vi "Analog multimeter producer-consumer.vi"() -> ()   [LabVIEW 2019]
uses:
  Controls/Enum_states.ctl
panel:
  in  "Output channel":T1(ring)
  in  "Input channel":T1(ring)
  in  "Data":bool
  in  "Settings":bool
  out "Message":string
  in  "Stop Button":bool
  out "Terminal GND":bool
  out "Terminal_I":bool
  out "Terminal_V":bool
  in  "Signal":dbl(knob) scale=0.0..1000.0
  in  "Zero instrument":dbl(knob) scale=-1.0..1.0
  in  "Zero resistance":dbl(knob) scale=-1.0..1.0
  in  "Selector":i32(knob)=10 min=0 max=20 step=1 scale=0.0..20.0
  out "Main indicator":dbl(knob) scale=0.0..1000.0
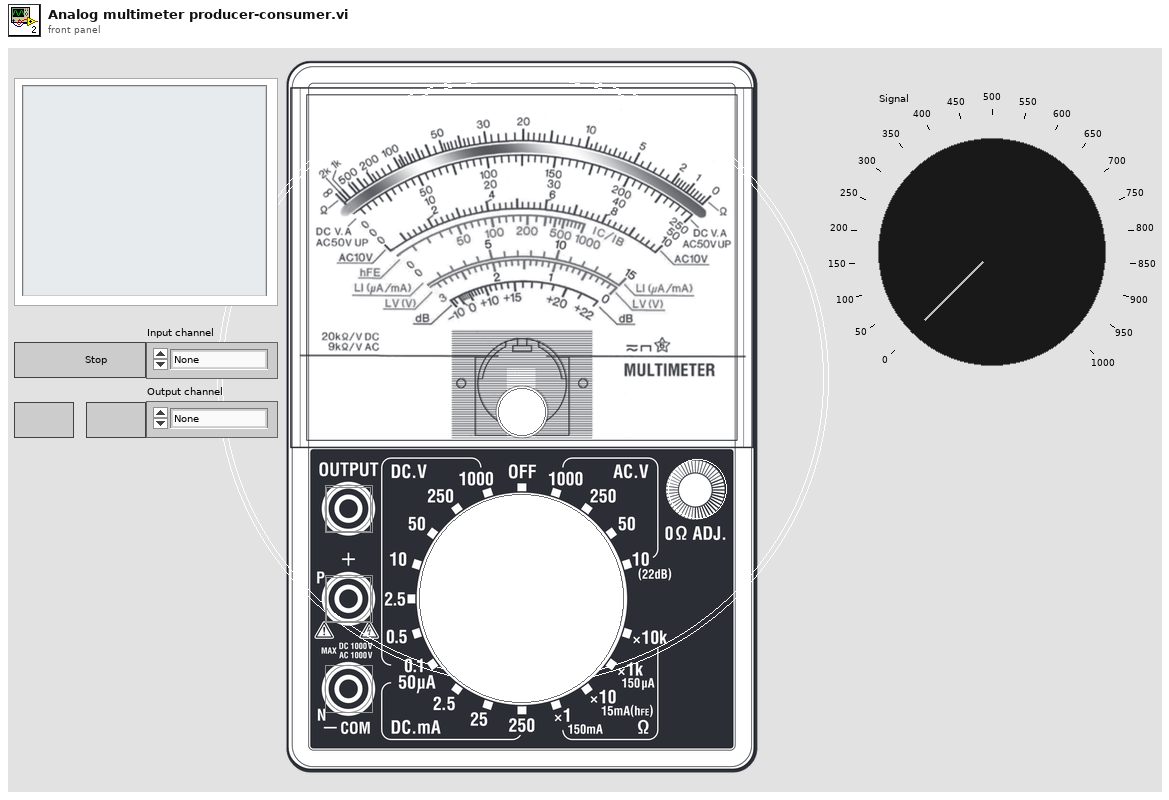
[diagram p1: front panel]
types:
  T1 = enum16{"None", "CH 1", "CH 2", "CH 3", "CH 4", "CH 5", ""}
  T2 = typedef "Enum_states.ctl" = enum16{"Initialize", "Run", "Load", "Stop"}
  T3 = cluster{"Main indicator":dbl, "Terminal_V":bool, "Terminal_I":bool, "Terminal GND":bool, "Message":string}
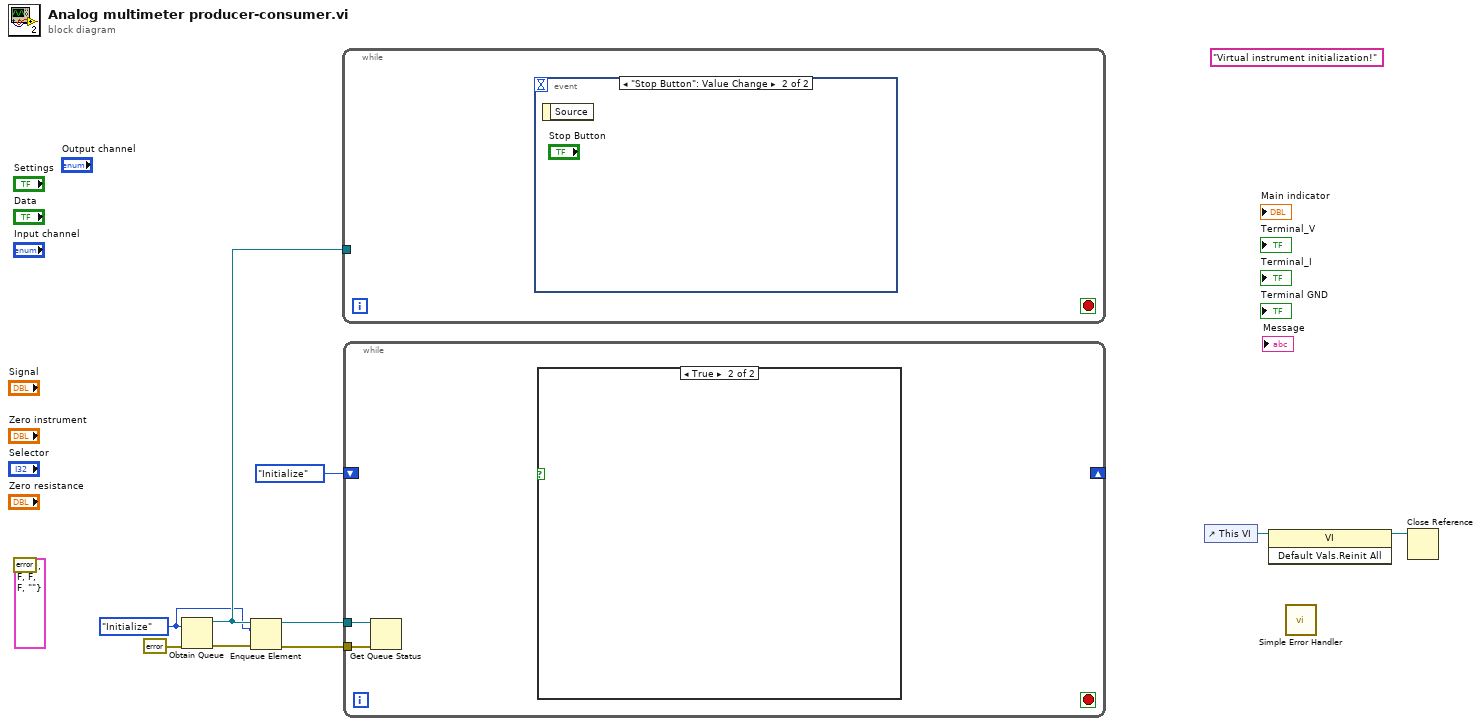
[diagram p0: block diagram]
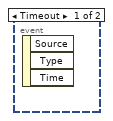
[diagram p3: hidden frame]
diagram:
  (unwired) "Virtual instrument initialization!" ("Message")
  w6 = Enum_states."Initialize" ("Enum")
  (unwired) T3 {"Main indicator"=0.0, "Terminal_V"=FALSE, "Terminal_I"=FALSE, "Terminal GND"=FALSE, "Message"=""}
  (unwired) errorcluster {"status"=FALSE, "code"=0, "source"=""} ("error constant")
  n1 = Obtain Queue(element data type=w6, error in (no error)=errorcluster {"status"=FALSE, "code"=0, "source"=""}) -> (queue out=w7:refnum<queue>, error out=w5:errorcluster)  [unwired: 3 in, 1 out]
  n2 = Enqueue Element(queue=w7, element=w6, error in (no error)=w5) -> (queue out=w3:refnum<queue>, error out=w2:errorcluster)  [unwired: 1 in, 1 out]
  n3 = while {
    tunnel: w7 -> [_]
    stop <- _ stop-if-true
    n4 = event shown="[1] \"Stop Button\": Value Change" {
      selector: _ -> [_ _]
      dyn-events: _ -> [_ _]
      timeout: _ -> [_ _]
      event Timeout {
        n5 = event-data() -> ()  [unwired: 1 in, 3 out]
      }
      event "Stop Button": Value Change {
        n6 = event-data() -> ()  [unwired: 1 in, 1 out]
      }
    }
  }
  n7 = while {
    shift-right: _ -> [_]
    shift-left: Enum_states."Initialize" ("Enum") -> [_]
    tunnel: w3 -> [w10]
    tunnel: w2 -> [w11]
    stop <- _ stop-if-true
    n8 = Get Queue Status(queue=w10, error in (no error)=w11) -> ()  [unwired: 1 in, 8 out]
    n9 = case shown="True" {
      selector: _ -> [_ _]
      frame False {
      }
      frame True {
      }
    }
  }
  n10 = control-ref of="This VI"() -> (w8:refnum<vi>)
  n11 = invoke class="VI" method="Default Vals.Reinit All"(reference=w8) -> (reference out=w9:refnum<vi>)  [unwired: 2 in, 2 out]
  n12 = call <vilib>:"Simple Error Handler.vi"() -> ()  [unwired: 5 in, 5 out]
  n13 = Close Reference(reference=w9) -> ()  [unwired: 1 in, 1 out]
